vi "Get 2D Plot Metadata.vi"(0 "Row Number":i32[](array[numeric]), 1 "Model?":bool, 5 "Source Location":i32[](array[numeric]), 7 "Interation number":i32, 9 "UVW index":i32[](array[numeric]), 11 "Scalar Value":dbl[](array[numeric]), 14 "Log Plot?":bool) -> (3 "Scalar limits":dbl[](array[numeric]), 4 "spreadsheet string":string, 6 "Max Min array":dbl[][](array[numeric]), 8 "Source Location":string, 10 "Data Directories":string[](array[string]), 12 "Wind Direction":dbl format="%0.2f", 15 "Stl Filename":string)   [LabVIEW 2020]
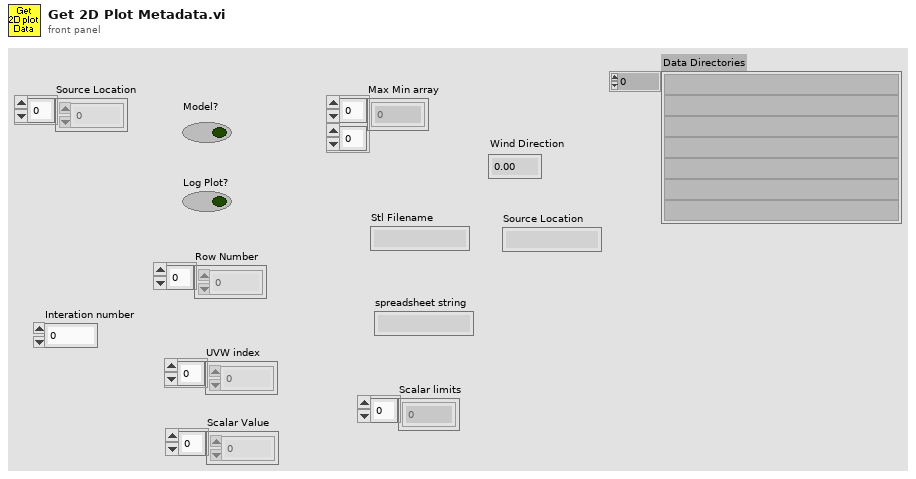
[diagram p1: front panel]
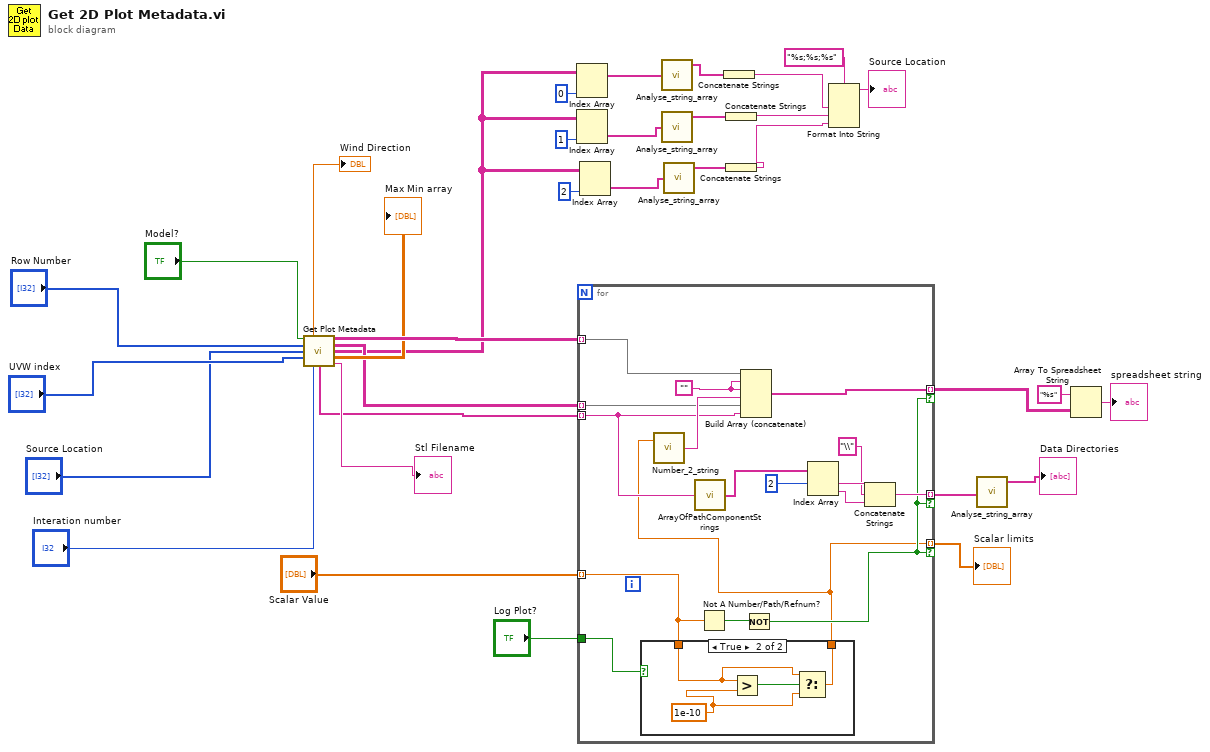
[diagram p0: block diagram]
diagram:
  n1 = call "Get Plot Metadata.vi"("Model?"="Model?", "Row Number"="Row Number", "Source Location"="Source Location", "UVW"="UVW index", "Interation number"="Interation number") -> ("Wind Direction"=→"Wind Direction":dbl, "Locations"=w28:string[][], "UVW"=w22:string[][], "Source Locations"=w15:string[][], "Max Min array"=→"Max Min array":dbl[][], "Raw Data Filenames"=w21:string[], "Stl Filename"=→"Stl Filename":string)  [unwired: 3 in, 1 out]
  n2 = Index Array(array=w15, index (col)=0 ("disabled index (col)")) -> (element=w14:string[])  [unwired: 1 in]
  n3 = Index Array(array=w15, index (col)=1 ("disabled index (col)")) -> (element=w12:string[])  [unwired: 1 in]
  n4 = for {
    tunnel: "Scalar Value" -> [w38] mode=indexing
    tunnel: [w35] -> w31 mode=indexing if=w36
    tunnel: "Log Plot?" -> [w51]
    tunnel: [w48] -> w32 mode=indexing if=w36
    tunnel: w22 -> [w47] mode=indexing
    tunnel: w28 -> [w46] mode=indexing
    tunnel: w21 -> [w40] mode=indexing
    tunnel: [w39] -> w2 mode=indexing if=w36
    w50 = ""
    n5 = case shown="True" w51 {
      tunnel: w38 -> [w52 w55]
      tunnel: [w52 w53] -> w35
      frame False {
      }
      frame True {
        w54 = 1e-10 ("y")
        n6 = Greater?(x=w55, y=w54) -> (0:w56:bool)
        n7 = Select(t=w55, s=w56, f=w54) -> (s? t:f=w53:dbl)
      }
    }
    n8 = call "Number_2_string.vi"("number"=w35) -> ("String"=w49:string)  [unwired: 1 in]
    n9 = call "ArrayOfPathComponentStrings.vi"("PathStringIn"=w40) -> ("ArrayOfPathComponentStringsOut"=w45:string[])
    n10 = Not A Number/Path/Refnum?(number/path/refnum=w38) -> (NaN/Path/Refnum?=w37:bool)
    n11 = Build Array (concatenate)(w46, w50, w50, w49, w47, w40) -> (w48:string[])
    n12 = Not(x=w37) -> (.not. x?=w36:bool)
    n13 = Index Array(array=w45, index #1=2 ("index")) -> (element #1=w43:string, element #2=w42:string)  [unwired: 1 in]
    n14 = Concatenate Strings(w43, "\\" ("string"), w42) -> (w39:string)
  }
  "Scalar limits" <- w31
  n15 = Index Array(array=w15, index (col)=2 ("disabled index (col)")) -> (element=w13:string[])  [unwired: 1 in]
  n16 = call "Analyse_string_array.vi"("String array"=w14) -> ("Unique strings"=w9:string[])  [unwired: 1 in, 1 out]
  n17 = call "Analyse_string_array.vi"("String array"=w12) -> ("Unique strings"=w10:string[])  [unwired: 1 in, 1 out]
  n18 = call "Analyse_string_array.vi"("String array"=w13) -> ("Unique strings"=w11:string[])  [unwired: 1 in, 1 out]
  n19 = Concatenate Strings(w9) -> (w8:string)
  n20 = Concatenate Strings(w10) -> (w7:string)
  n21 = Concatenate Strings(w11) -> (w6:string)
  n22 = Format Into String(format string="%s;%s;%s", w8, w7, w6) -> (resulting string=→"Source Location":string)  [unwired: 2 in, 1 out]
  n23 = call "Analyse_string_array.vi"("String array"=w2) -> ("Unique strings"=→"Data Directories":string[])  [unwired: 1 in, 1 out]
  n24 = Array To Spreadsheet String(array=w32, 3:"%s" ("format string")) -> (spreadsheet string=→"spreadsheet string":string)  [unwired: 1 in]
